vi "remove_csv_header.vi"(2 "first row":dbl[](array[numeric]), 3 "all rows":dbl[][](array[numeric])) -> (0 "deleted portion":dbl[][](array[numeric]), 1 "array w/ subset deleted":dbl[][](array[numeric]))   [LabVIEW 2011]
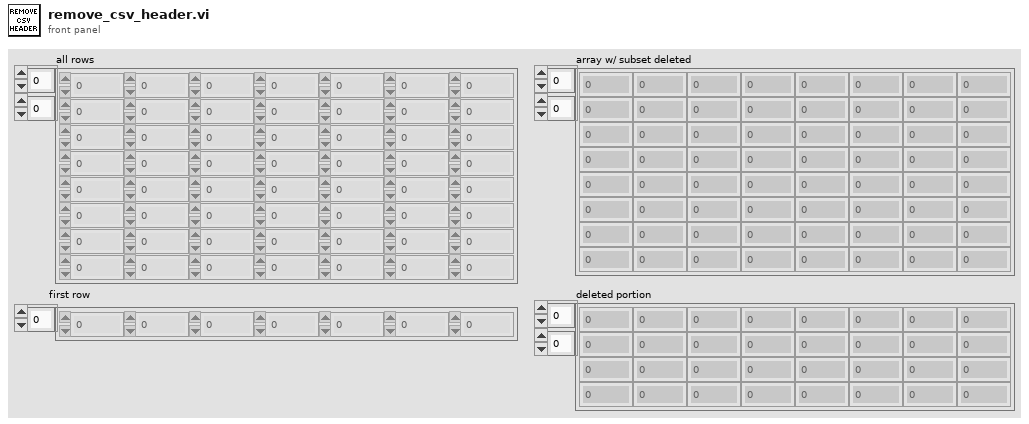
[diagram p1: front panel]
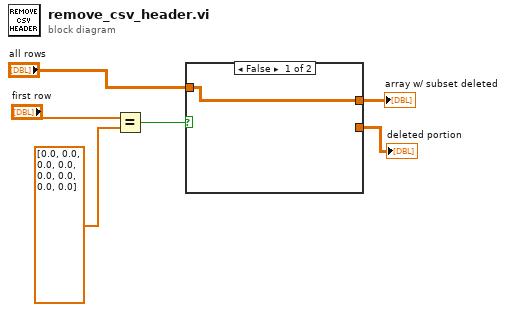
[diagram p0: block diagram]
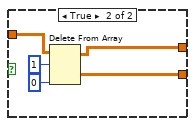
[diagram p2: hidden frame]
diagram:
  n1 = Equal?(x="first row", y=dbl[] [0.0, 0.0, 0.0, 0.0, 0.0, 0.0, 0.0, 0.0]) -> (x = y?=w5:bool)
  n2 = case shown="False" w5 {
    tunnel: "all rows" -> [w7 w10]
    tunnel: [_ w9] -> w4
    tunnel: [w7 w8] -> w3
    frame False {
    }
    frame True {
      n3 = Delete From Array(array=w10, length=1, index (row)=0 ("index")) -> (deleted portion=w9:dbl[][], array with subset deleted=w8:dbl[][])  [unwired: 1 in]
    }
  }
  "array w/ subset deleted" <- w3
  "deleted portion" <- w4
